vi "S4GUI.vi"(7 "Tab ObsEng":enum32{"Obs", "CCD modes", "Guider", "Eng"}(tab)) -> ()   [LabVIEW 2018] (continued)
            n1225 = call "Read Instrument.lvclass.vi"("error in (no error)"=w304, "S4ACS_GUI in"=w306) -> ("error out"=w308:errorcluster, "Instrument.lvclass"=w307:refnum<class "Instrument.lvclass">, "S4ACS_GUI out"=w296:refnum<class "S4GUI.lvclass">)  [unwired: 7 in]
            n1226 = call-dynamic "Read mode.vi"("error in (no error)"=w308, "Instrument in"=w307) -> ("error out"=w297:errorcluster, "mode"=w309:bool)  [unwired: 7 in, 1 out]
            n1227 = while {
              tunnel: w309 -> [w351]
              shift-right: [w347] -> _
              shift-left: _ -> [w350]
              shift-right: [w348] -> _
              shift-left: _ -> [w349]
              stop <- TRUE stop-if-true
              n1228 = case shown="False" w351 {
                tunnel: w350 -> [w353 w372]
                tunnel: [w354 w371] -> w347
                tunnel: w349 -> [w356 w370]
                tunnel: [w355 w369] -> w348
                frame True {
                  # "polarimetria"
                  n1229 = case shown="False" w356 {
                    selector: w356 -> [w366 w368]
                    tunnel: [w365 w368] -> w355
                    tunnel: [FALSE FALSE] -> w354
                    tunnel: w353 -> [_ _]
                    frame False {
                      w363 = 11
                      w360 = 80
                      w359 = 12900
                      # "Valor médio\ndo curso do foco."
                      n1230 = local write "Start focus"(w359) -> ()
                      n1231 = local write "Step focus"(w360) -> ()
                      n1232 = local write "#steps"(w363) -> ()
                      n1233 = Quotient & Remainder(x=w363, y=2) -> (floor(x/y)=w361:i32)  [unwired: 1 out]
                      n1234 = Multiply(x=w360, y=w361) -> (x*y=w358:i32)
                      n1235 = Add(x=w359, y=w358) -> (x+y=w357:i32)
                      n1236 = local write "Target focus 2"(w357) -> ()
                      n1237 = local write "Target focus"(w357) -> ()
                      n1238 = Not(x=w366) -> (.not. x?=w365:bool)
                    }
                    frame True {
                    }
                  }
                }
                frame False {
                  # "fotometria"
                  n1239 = case shown="False" w372 {
                    selector: w372 -> [w381 w384]
                    tunnel: [w380 w384] -> w371
                    tunnel: w370 -> [_ _]
                    tunnel: [FALSE FALSE] -> w369
                    frame False {
                      w376 = 11
                      w375 = 100
                      w374 = 13400
                      # "Valor médio\ndo curso do foco."
                      n1240 = local write "Start focus"(w374) -> ()
                      n1241 = local write "Step focus"(w375) -> ()
                      n1242 = local write "#steps"(w376) -> ()
                      n1243 = Quotient & Remainder(x=w376, y=2) -> (floor(x/y)=w378:i32)  [unwired: 1 out]
                      n1244 = Multiply(x=w375, y=w378) -> (x*y=w377:i32)
                      n1245 = Add(x=w374, y=w377) -> (x+y=w373:i32)
                      n1246 = local write "Target focus"(w373) -> ()
                      n1247 = local write "Target focus 2"(w373) -> ()
                      n1248 = Not(x=w381) -> (.not. x?=w380:bool)
                    }
                    frame True {
                    }
                  }
                }
              }
            }
            n1249 = call-dynamic "Read exit.vi"("error in (no error)"=w297, "S4GUI in"=w296) -> ("error out"=w295:errorcluster, "exit"=w294:bool, "S4GUI out"=w293:refnum<class "S4GUI.lvclass">)  [unwired: 7 in]
          }
        }
      }
      event "Lambda Selector": Mouse Down? {
        n1250 = event-data() -> ()  [unwired: 1 in, 7 out]
        n1251 = First Call?() -> (First Call?: T/F=w2000:bool)
        n1252 = case shown="True" w2000 {
          tunnel: w2002 -> [w2004 w2006]
          tunnel: [w2004 w2005] -> w2001
          frame False {
          }
          frame True {
            w2008 = u16 0 items=["OFF", "Lambda/2", "Lambda/4"] ("Lambda Selector")
            n1253 = property on="Lambda Selector" class="Ring (strict)"(error in=w2006, "Value"=w2008) -> (error out=w2009:errorcluster)  [unwired: 1 in, 1 out]
            n1254 = property on="Lambda Selector" class="Ring (strict)"(error in=w2009, "RingText.Text"="OFF" ("Boolean Text.Text")) -> (error out=w2005:errorcluster)  [unwired: 1 in, 1 out]
          }
        }
        n1255 = event-data() -> ()  [unwired: 2 in, 1 out]
      }
      event "object suffix": Key Down; "object suffix": Key Repeat {
        n1256 = event-data() -> ("Char"=w2010:i16)  [unwired: 1 in]
        "charKeyboardInteger" <- w2010
        n1257 = call-dynamic "Write charSuffix.vi"("error in (no error)"=w2013, "charSuffix"=w2010, "S4GUI in"=w2014) -> ("error out"=w2011:errorcluster, "S4GUI out"=w2012:refnum<class "S4GUI.lvclass">)  [unwired: 7 in]
      }
      event "dflat suffix": Key Down; "dflat suffix": Key Repeat {
        n1258 = event-data() -> ("Char"=w2017:i16)  [unwired: 1 in]
        n1259 = call-dynamic "Write charSuffix.vi"("error in (no error)"=w2018, "charSuffix"=w2017, "S4GUI in"=w2019) -> ("error out"=w2015:errorcluster, "S4GUI out"=w2016:refnum<class "S4GUI.lvclass">)  [unwired: 7 in]
      }
      event "sflat suffix": Key Down; "sflat suffix": Key Repeat {
        n1260 = event-data() -> ("Char"=w2022:i16)  [unwired: 1 in]
        n1261 = call-dynamic "Write charSuffix.vi"("error in (no error)"=w2023, "charSuffix"=w2022, "S4GUI in"=w2024) -> ("error out"=w2020:errorcluster, "S4GUI out"=w2021:refnum<class "S4GUI.lvclass">)  [unwired: 7 in]
      }
      event "dark suffix": Key Down; "dark suffix": Key Repeat {
        n1262 = event-data() -> ("Char"=w2027:i16)  [unwired: 1 in]
        n1263 = call-dynamic "Write charSuffix.vi"("error in (no error)"=w2028, "charSuffix"=w2027, "S4GUI in"=w2029) -> ("error out"=w2025:errorcluster, "S4GUI out"=w2026:refnum<class "S4GUI.lvclass">)  [unwired: 7 in]
      }
      event "zero suffix": Key Down; "zero suffix": Key Repeat {
        n1264 = event-data() -> ("Char"=w2032:i16)  [unwired: 1 in]
        n1265 = call-dynamic "Write charSuffix.vi"("error in (no error)"=w2033, "charSuffix"=w2032, "S4GUI in"=w2034) -> ("error out"=w2030:errorcluster, "S4GUI out"=w2031:refnum<class "S4GUI.lvclass">)  [unwired: 7 in]
      }
      event "focus suffix": Key Down; "focus suffix": Key Repeat {
        n1266 = event-data() -> ("Char"=w2037:i16)  [unwired: 1 in]
        n1267 = call-dynamic "Write charSuffix.vi"("error in (no error)"=w2038, "charSuffix"=w2037, "S4GUI in"=w2039) -> ("error out"=w2035:errorcluster, "S4GUI out"=w2036:refnum<class "S4GUI.lvclass">)  [unwired: 7 in]
      }
      event "Set CCD mode": Value Change {
        w2152 = i16 1 items=["Cooler OFF", "Cooler ON"] ("Cooler ON/OFF")
        w2166 = i16 1 items=["Cooler OFF", "Cooler ON"] ("Cooler ON/OFF")
        w2182 = i16 1 items=["Cooler OFF", "Cooler ON"] ("Cooler ON/OFF")
        w2202 = i16 1 items=["Cooler OFF", "Cooler ON"] ("Cooler ON/OFF")
        # "Sinaliza que houve requisição de SET CCD mode"
        n1268 = event-data() -> ()  [unwired: 1 in, 6 out]
        n1269 = call-dynamic "Write User Event.vi"("error in (no error)"=w2358, "User Event"="SET CCD mode ", "S4GUI in"=w2357) -> ("error out"=w2147:errorcluster, "S4GUI out"=w2146:refnum<class "S4GUI.lvclass">)  [unwired: 7 in]
        n1270 = call-dynamic "Write SET request.vi"("error in (no error)"=w2147, "SET request"=TRUE, "S4GUI in"=w2146) -> ("error out"=w2144:errorcluster, "S4GUI out"=w2145:refnum<class "S4GUI.lvclass">)  [unwired: 7 in]
        n1271 = call-dynamic "Read CCD mode.vi"("error in (no error)"=w2144, "S4GUI in"=w2145) -> ("error out"=w2355:errorcluster, "CCD mode"=w2356:T30, "S4GUI out"=w2354:refnum<class "S4GUI.lvclass">)  [unwired: 7 in]
        n1272 = Bundle By Name(cluster=w2356, "FTM"="Frame Transfer", "AQM"="AQM", "SZM"="SZM", "EM gain"="EM Gain") -> (w2353:T30)
        n1273 = call-dynamic "Write CCD mode.vi"("error in (no error)"=w2355, "CCD mode"=w2353, "S4GUI in"=w2354) -> ("error out"=w2213:errorcluster, "S4GUI out"=w2214:refnum<class "S4GUI.lvclass">)  [unwired: 7 in]
        n1274 = call-dynamic "LoadCCDmode.vi"("error in (no error)"=w2213, "S4GUI in"=w2214) -> ("error out"=w2212:errorcluster, "S4GUI out"=w2211:refnum<class "S4GUI.lvclass">)  [unwired: 8 in]
        n1275 = call-dynamic "Read Parameters CCD modes.vi"("error in (no error)"=w2212, "S4GUI in"=w2211) -> ("error out"=w2210:errorcluster, "Parameters CCD modes"=w2215:T5, "S4GUI out"=w2209:refnum<class "S4GUI.lvclass">)  [unwired: 7 in]
        n1276 = Unbundle By Name(w2215) -> ("CCD \nEM Mode"=w2345:u8, "Readout\nRate"=w2207:u8)
        n1277 = case shown="0, Default" w2345 {
          tunnel: [string[] ["30 MHz", "20 MHz", "10 MHz", "1 MHz"] ("Strings []") string[] ["1 MHz", "0.1 MHz"] ("Strings []")] -> w2346
          frame 0, Default {
          }
          frame 1 {
          }
        }
        n1278 = flat-sequence {
          tunnel: w2346 -> [w2492]
          tunnel: w2345 -> [w2493]
          tunnel: [w2493] -> w2347
          tunnel: w2215 -> [w2499]
          tunnel: [w2498] -> w2208
          tunnel: w2347 -> [w2496]
          tunnel: w2216 -> [w2497]
          tunnel: w2207 -> [w2494]
          frame #0 {
            n1279 = property on="Readout\nRate" class="Ring (strict)"("Strings []"=w2492) -> ()  [unwired: 2 in, 2 out]
            n1280 = property on="Readout\nRate" class="Ring (strict)"("Strings []"=w2492) -> ()  [unwired: 2 in, 2 out]
            n1281 = property on="Readout Rate 2" class="Ring (strict)"("Strings []"=w2492) -> ()  [unwired: 2 in, 2 out]
            n1282 = property on="Readout Rate" class="Ring (strict)"("Strings []"=w2492) -> ()  [unwired: 2 in, 2 out]
            n1283 = property on="Readout Rate 3" class="Ring (strict)"("Strings []"=w2492) -> ()  [unwired: 2 in, 2 out]
            n1284 = property on="Readout Rate 4" class="Ring (strict)"("Strings []"=w2492) -> ()  [unwired: 2 in, 2 out]
          }
          frame #1 {
            n1285 = Bundle By Name(cluster=w2499, "Readout\nRate"=w2494, "CCD \nEM Mode"=w2496) -> (w2498:T5)
            n1286 = disable-structure shown="Enabled" {
              disable-tunnel: w2497 -> [w2503 w2504]
              disable-tunnel: w2496 -> [w2502 _]
              disable-tunnel: [w2501 w2504] -> w2495
              disable-tunnel: w2494 -> [w2500 _]
              frame Disabled {
                n1287 = Bundle By Name(cluster=w2503, "Parameters.Readout\nRate"=w2500, "Parameters.CCD \nEM Mode"=w2502) -> (w2501:T8)
              }
              frame Enabled {
              }
            }
            n1288 = local write "Input Cluster"(w2495) -> ()
          }
        }
        n1289 = call-dynamic "Read InfoCCDmode.vi"("error in (no error)"=w2210, "S4GUI in"=w2209) -> ("error out"=w2348:errorcluster, "InfoCCDmode"=w2077:T2, "S4GUI out"=w2349:refnum<class "S4GUI.lvclass">)  [unwired: 7 in]
        "InfoCCDmode" <- w2077
        n1290 = Unbundle By Name(w2077) -> ("MinExpTime"=w2099:dbl)
        n1291 = call-dynamic "Read Parameters CCD modes.vi"("error in (no error)"=w2348, "S4GUI in"=w2349) -> ("error out"=w2342:errorcluster, "Parameters CCD modes"=→"Parameters CCD modes":T5, "S4GUI out"=w2343:refnum<class "S4GUI.lvclass">)  [unwired: 7 in]
        n1292 = local read "Input Cluster"() -> (w2216:T8)
        n1293 = call-dynamic "Write Parameters CCD modes.vi"("error in (no error)"=w2342, "Parameters CCD modes"=w2208, "S4GUI in"=w2343) -> ("error out"=w2321:errorcluster, "S4GUI out"=w2295:refnum<class "S4GUI.lvclass">)  [unwired: 7 in]
        n1294 = Unbundle By Name(w2208) -> ("Frame\nTransfer"=w2250:bool, "Pre-amplification\nGain"=w2249:u8, "Readout\nRate"=w2248:u8, "CCD \nEM Mode"=w2247:u8, "CCD\nEM Gain"=w2246:u16, "Image \nInitial Line"=w2245:u16, "Image\nInitial Column"=w2244:u16, "Image\nFinal Line"=w2234:u16, "Image\nFInal Column"=w2243:u16, "Vertical\nBinning"=w2242:u16, "Horizontal\nBinning"=w2241:u16)
        n1295 = call-dynamic "Read AcquisitionA.vi"("error in (no error)"=w2321, "S4ACS_GUI in"=w2295) -> ("error out"=w2232:errorcluster, "Acquisition.lvclass"=w2233:refnum<class "Acquisition.lvclass">, "S4ACS_GUI out"=w2341:refnum<class "S4GUI.lvclass">)  [unwired: 7 in]
        n1296 = call-dynamic "Read enabled.vi"("error in (no error)"=w2232, "Server in"=w2233) -> ("error out"=w2231:errorcluster, "enabled"=w2229:bool, "Server out"=w2230:refnum<class "Acquisition.lvclass">)  [unwired: 7 in]
        n1297 = call-dynamic "Read Channel.vi"("error in (no error)"=w2231, "Acquisition in"=w2230) -> ("error out"=w2338:errorcluster, "Channel.lvclass"=w2339:refnum<class "Channel.lvclass">, "Acquisition out"=w2340:refnum<class "Acquisition.lvclass">)  [unwired: 7 in]
        n1298 = call-dynamic "Read Interface.vi"("error in (no error)"=w2338, "Channel in"=w2339) -> ("error out"=w2324:errorcluster, "Interface.lvclass"=w2325:refnum<class "Interface.lvclass">, "Channel out"=w2319:refnum<class "Channel.lvclass">)  [unwired: 7 in]
        n1299 = call-dynamic "Write PREV_FT.vi"("error in (no error)"=w2324, "PREV_FT"=w2250, "Interface in"=w2325) -> ("error out"=w2205:errorcluster, "Interface out"=w2204:refnum<class "Interface.lvclass">)  [unwired: 7 in]
        n1300 = call-dynamic "Write Cooler ON_OFF.vi"("error in (no error)"=w2205, "Cooler ON/OFF"=w2202, "Interface in"=w2204) -> ("error out"=w2203:errorcluster, "Interface out"=w2201:refnum<class "Interface.lvclass">)  [unwired: 7 in]
        n1301 = call-dynamic "Read target cluster.vi"("error in (no error)"=w2203, "Channel in"=w2319) -> ("error out"=w2317:errorcluster, "target cluster"=w2316:T31, "Channel out"=w2318:refnum<class "Channel.lvclass">)  [unwired: 7 in]
        n1302 = Bundle By Name(cluster=w2316, "FRAME_TRANSFER"=w2250, "PREAMP"=w2249, "READOUT_RATE"=w2248, "EM_MODE"=w2247, "EM_GAIN"=w2246, "INITIAL_LINE"=w2245, "INITIAL_COLUMN"=w2244, "FINAL_LINE"=w2234, "FINAL_COLUMN"=w2243, "VBIN"=w2242, "HBIN"=w2241) -> (w2198:T31)
        n1303 = call-dynamic "Write target cluster.vi"("error in (no error)"=w2317, "target cluster"=w2198, "Channel in"=w2318) -> ("error out"=w2199:errorcluster, "Channel out"=w2323:refnum<class "Channel.lvclass">)  [unwired: 7 in]
        n1304 = call-dynamic "Set CCD_Config.vi"("error in (no error)"=w2199, "input cluster"=w2198, "Interface in"=w2201) -> ("error out"=w2188:errorcluster, "Interface out"=w2200:refnum<class "Interface.lvclass">)  [unwired: 7 in]
        n1305 = Flatten To String(anything=w2198, error in (no error)=w2199) -> (data string=w2333:string)  [unwired: 2 in, 2 out]
        n1306 = call "Write flatted cluster.vi"("error in (no error)"=w2188, "flatted cluster"=w2333, "Interface in"=w2200) -> ("error out"=w2138:errorcluster, "Interface out"=w2139:refnum<class "Interface.lvclass">)  [unwired: 7 in]
        n1307 = call "Read Exposure Time.vi"("error in (no error)"=w2138, "Interface in"=w2139) -> ("error out"=w2136:errorcluster, "Exposure Time"=w2141:dbl, "Interface out"=w2137:refnum<class "Interface.lvclass">)  [unwired: 7 in]
        n1308 = Greater Or Equal?(x=w2141, y=w2099) -> (x >= y?=w2142:bool)
        n1309 = Select(t=w2141, s=w2142, f=w2099) -> (s? t:f=w2140:dbl)
        n1310 = local write "Exptime ch1"(w2140) -> ()
        n1311 = call "Write Exposure Time.vi"("error in (no error)"=w2136, "Exposure Time"=w2140, "Interface in"=w2137) -> ("error out"=w2097:errorcluster, "Interface out"=w2098:refnum<class "Interface.lvclass">)  [unwired: 7 in]
        n1312 = call-dynamic "ValidateExp.vi"("error in (no error)"=w2097, "Interface in"=w2098) -> ("error out"=w2080:errorcluster, "Interface out"=w2082:refnum<class "Interface.lvclass">)  [unwired: 8 in]
        n1313 = call-dynamic "Read MAX #FRAMES.vi"("error in (no error)"=w2080, "Interface in"=w2082) -> ("error out"=w2079:errorcluster, "MAX #FRAMES"=w2076:u32, "Interface out"=w2081:refnum<class "Interface.lvclass">)  [unwired: 7 in]
        n1314 = call-dynamic "Read # Images.vi"("error in (no error)"=w2079, "Interface in"=w2081) -> ("error out"=w2095:errorcluster, "# Images"=w2083:u32, "Interface out"=w2096:refnum<class "Interface.lvclass">)  [unwired: 7 in]
        n1315 = call-dynamic "Write #PREV Images.vi"("error in (no error)"=w2095, "#PREV FRAMES"=w2083, "Interface in"=w2096) -> ("error out"=w2093:errorcluster, "Interface out"=w2094:refnum<class "Interface.lvclass">)  [unwired: 7 in]
        n1316 = call-dynamic "Write Interface.vi"("error in (no error)"=w2093, "Interface.lvclass"=w2094, "Channel in"=w2323) -> ("error out"=w2329:errorcluster, "Channel out"=w2331:refnum<class "Channel.lvclass">)  [unwired: 7 in]
        n1317 = local write "Exp ch1"(w2083) -> ()
        n1318 = property on="Exposures Done ch1" class="Slide (strict)"("Scale.Maximum"=w2083, "Scale.Minimum"=0.0 ("Scale.Range:Minimum")) -> ()  [unwired: 2 in, 2 out]
        n1319 = call "Write section_name.vi"("error in (no error)"=w2329, "section_name"="CCD_ACS1", "Channel in"=w2331) -> ("error out"=w2328:errorcluster, "Channel out"=w2330:refnum<class "Channel.lvclass">)  [unwired: 7 in]
        n1320 = call-dynamic "save config.vi"("error in (no error)"=w2328, "file config"="lastsaved.cfg", "Channel in"=w2330) -> ("error out"=w2196:errorcluster, "Channel out"=w2197:refnum<class "Channel.lvclass">)  [unwired: 7 in]
        n1321 = call-dynamic "ValidateConfig.vi"("error in (no error)"=w2196, "Channel in"=w2197) -> ("error out"=w2194:errorcluster, "Channel out"=w2195:refnum<class "Channel.lvclass">)  [unwired: 7 in, 1 out]
        n1322 = call-dynamic "Save Temp.vi"("error in (no error)"=w2194, "temp file"="lasttemp.cfg" ("file config"), "Channel in"=w2195) -> ("error out"=w2193:errorcluster, "Channel out"=w2192:refnum<class "Channel.lvclass">)  [unwired: 7 in]
        n1323 = case shown="True" w2229 {
          tunnel: [w2460 w2485] -> w2337
          tunnel: [w2459 w2484] -> w2336
          tunnel: w2192 -> [w2460 w2483]
          tunnel: w2193 -> [w2459 w2482]
          frame False {
          }
          frame True {
            # "Esvazia\na fila."
            n1324 = call-dynamic "Read State Machine.vi"("error in (no error)"=w2482, "Device in"=w2483) -> ("error out"=w2476:errorcluster, "State Machine.lvclass"=w2479:refnum<class "State Machine.lvclass">, "Device out"=w2489:refnum<class "Channel.lvclass">)  [unwired: 7 in]
            n1325 = call-dynamic "Read ref StatesQueue.vi"("error in (no error)"=w2476, "State Machine in"=w2479) -> ("error out"=w2467:errorcluster, "ref StatesQueue"=w2469:refnum<queue>, "State Machine out"=w2478:refnum<class "State Machine.lvclass">)  [unwired: 7 in]
            n1326 = Flush Queue(queue=w2469, error in (no error)=w2467) -> (queue out=w2468:refnum<queue>, error out=w2466:errorcluster)  [unwired: 1 out]
            n1327 = Enqueue Element(queue=w2468, element=u32 60 ("State"), error in (no error)=w2466) -> (queue out=w2481:refnum<queue>, error out=w2475:errorcluster)  [unwired: 1 in, 1 out]
            n1328 = Enqueue Element(queue=w2481, element=u32 45 ("State"), error in (no error)=w2475) -> (queue out=w2480:refnum<queue>, error out=w2474:errorcluster)  [unwired: 1 in, 1 out]
            n1329 = Enqueue Element(queue=w2480, element=u32 35 ("State"), error in (no error)=w2474) -> (queue out=w2464:refnum<queue>, error out=w2463:errorcluster)  [unwired: 1 in, 1 out]
            n1330 = Enqueue Element(queue=w2464, element=u32 37 ("State"), error in (no error)=w2463) -> (queue out=w2461:refnum<queue>, error out=w2462:errorcluster)  [unwired: 1 in, 1 out]
            n1331 = call-dynamic "Write ref StatesQueue.vi"("error in (no error)"=w2462, "ref StatesQueue"=w2461, "State Machine in"=w2478) -> ("error out"=w2470:errorcluster, "State Machine out"=w2477:refnum<class "State Machine.lvclass">)  [unwired: 7 in]
            n1332 = disable-structure shown="Enabled" {
              disable-tunnel: [0 ("State") 45] -> w2486
              frame Enabled {
                # "Vai pra 0 para que\nos estados da fila \nsejam retirados."
              }
              frame Disabled {
                # "Verifica Texp\nantes de tudo."
              }
            }
            n1333 = call-dynamic "Write State.vi"("error in (no error)"=w2470, "State"=w2486, "State Machine in"=w2477) -> ("error out"=w2487:errorcluster, "State Machine out"=w2488:refnum<class "State Machine.lvclass">)  [unwired: 7 in]
            n1334 = call-dynamic "Write State Machine.vi"("error in (no error)"=w2487, "State Machine.lvclass"=w2488, "Device in"=w2489) -> ("error out"=w2484:errorcluster, "Device out"=w2485:refnum<class "Channel.lvclass">)  [unwired: 7 in]
          }
        }
        n1335 = Bundle By Name(cluster=w2077, "MaxExp"=w2076) -> (w2078:T2)
        n1336 = call-dynamic "Write Channel.vi"("error in (no error)"=w2336, "Channel.lvclass"=w2337, "Acquisition in"=w2340) -> ("error out"=w2335:errorcluster, "Acquisition out"=w2334:refnum<class "Acquisition.lvclass">)  [unwired: 7 in]
        n1337 = local write "InfoCCDmode"(w2078) -> ()
        n1338 = call-dynamic "Write AcquisitionA.vi"("error in (no error)"=w2335, "Acquisition.lvclass"=w2334, "S4ACS_GUI in"=w2341) -> ("error out"=w2090:errorcluster, "S4ACS_GUI out"=w2091:refnum<class "S4GUI.lvclass">)  [unwired: 7 in]
        n1339 = call-dynamic "Read InfoCCDmode.vi"("error in (no error)"=w2090, "S4GUI in"=w2091) -> ("error out"=w2088:errorcluster, "InfoCCDmode"=w2087:T2, "S4GUI out"=w2089:refnum<class "S4GUI.lvclass">)  [unwired: 7 in]
        n1340 = Bundle By Name(cluster=w2087, "MaxExp"=w2076) -> (w2086:T2)
        n1341 = call-dynamic "Write InfoCCDmode.vi"("error in (no error)"=w2088, "InfoCCDmode"=w2086, "S4GUI in"=w2089) -> ("error out"=w2084:errorcluster, "S4GUI out"=w2085:refnum<class "S4GUI.lvclass">)  [unwired: 7 in]
        n1342 = call "Read AcquisitionB.vi"("error in (no error)"=errorcluster {"status"=FALSE, "code"=0, "source"=""}, "S4ACS_GUI in"=w2085) -> ("error out"=w2225:errorcluster, "Acquisition.lvclass"=w2228:refnum<class "Acquisition.lvclass">, "S4ACS_GUI out"=w2315:refnum<class "S4GUI.lvclass">)  [unwired: 7 in]
        n1343 = call-dynamic "Read enabled.vi"("error in (no error)"=w2225, "Server in"=w2228) -> ("error out"=w2226:errorcluster, "enabled"=w2121:bool, "Server out"=w2227:refnum<class "Acquisition.lvclass">)  [unwired: 7 in]
        n1344 = call-dynamic "Read Channel.vi"("error in (no error)"=w2226, "Acquisition in"=w2227) -> ("error out"=w2312:errorcluster, "Channel.lvclass"=w2313:refnum<class "Channel.lvclass">, "Acquisition out"=w2314:refnum<class "Acquisition.lvclass">)  [unwired: 7 in]
        n1345 = call-dynamic "Read Interface.vi"("error in (no error)"=w2312, "Channel in"=w2313) -> ("error out"=w2301:errorcluster, "Interface.lvclass"=w2302:refnum<class "Interface.lvclass">, "Channel out"=w2299:refnum<class "Channel.lvclass">)  [unwired: 7 in]
        n1346 = call-dynamic "Write PREV_FT.vi"("error in (no error)"=w2301, "PREV_FT"=w2250, "Interface in"=w2302) -> ("error out"=w2183:errorcluster, "Interface out"=w2185:refnum<class "Interface.lvclass">)  [unwired: 7 in]
        n1347 = call-dynamic "Write Cooler ON_OFF.vi"("error in (no error)"=w2183, "Cooler ON/OFF"=w2182, "Interface in"=w2185) -> ("error out"=w2181:errorcluster, "Interface out"=w2184:refnum<class "Interface.lvclass">)  [unwired: 7 in]
        n1348 = call-dynamic "Read target cluster.vi"("error in (no error)"=w2181, "Channel in"=w2299) -> ("error out"=w2297:errorcluster, "target cluster"=w2296:T31, "Channel out"=w2298:refnum<class "Channel.lvclass">)  [unwired: 7 in]
        n1349 = Bundle By Name(cluster=w2296, "FRAME_TRANSFER"=w2250, "PREAMP"=w2249, "READOUT_RATE"=w2248, "EM_MODE"=w2247, "EM_GAIN"=w2246, "INITIAL_LINE"=w2245, "INITIAL_COLUMN"=w2244, "FINAL_LINE"=w2234, "FINAL_COLUMN"=w2243, "VBIN"=w2242, "HBIN"=w2241) -> (w2186:T31)
        n1350 = call-dynamic "Write target cluster.vi"("error in (no error)"=w2297, "target cluster"=w2186, "Channel in"=w2298) -> ("error out"=w2189:errorcluster, "Channel out"=w2300:refnum<class "Channel.lvclass">)  [unwired: 7 in]
        n1351 = call-dynamic "Set CCD_Config.vi"("error in (no error)"=w2189, "input cluster"=w2186, "Interface in"=w2184) -> ("error out"=w2187:errorcluster, "Interface out"=w2190:refnum<class "Interface.lvclass">)  [unwired: 7 in]
        n1352 = Flatten To String(anything=w2186, error in (no error)=w2189) -> (data string=w2309:string)  [unwired: 2 in, 2 out]
        n1353 = call "Write flatted cluster.vi"("error in (no error)"=w2187, "flatted cluster"=w2309, "Interface in"=w2190) -> ("error out"=w2114:errorcluster, "Interface out"=w2115:refnum<class "Interface.lvclass">)  [unwired: 7 in]
        n1354 = call "Read Exposure Time.vi"("error in (no error)"=w2114, "Interface in"=w2115) -> ("error out"=w2135:errorcluster, "Exposure Time"=w2116:dbl, "Interface out"=w2134:refnum<class "Interface.lvclass">)  [unwired: 7 in]
        n1355 = Greater Or Equal?(x=w2116, y=w2099) -> (x >= y?=w2132:bool)
        n1356 = Select(t=w2116, s=w2132, f=w2099) -> (s? t:f=w2133:dbl)
        n1357 = local write "Exptime ch2"(w2133) -> ()
        n1358 = call "Write Exposure Time.vi"("error in (no error)"=w2135, "Exposure Time"=w2133, "Interface in"=w2134) -> ("error out"=w2061:errorcluster, "Interface out"=w2066:refnum<class "Interface.lvclass">)  [unwired: 7 in]
        n1359 = call-dynamic "ValidateExp.vi"("error in (no error)"=w2061, "Interface in"=w2066) -> ("error out"=w2074:errorcluster, "Interface out"=w2065:refnum<class "Interface.lvclass">)  [unwired: 8 in]
        n1360 = call-dynamic "Read MAX #FRAMES.vi"("error in (no error)"=w2074, "Interface in"=w2065) -> ("error out"=w2075:errorcluster, "Interface out"=w2064:refnum<class "Interface.lvclass">)  [unwired: 7 in, 1 out]
        n1361 = call-dynamic "Read # Images.vi"("error in (no error)"=w2075, "Interface in"=w2064) -> ("error out"=w2073:errorcluster, "# Images"=w2058:u32, "Interface out"=w2063:refnum<class "Interface.lvclass">)  [unwired: 7 in]
        n1362 = call-dynamic "Write #PREV Images.vi"("error in (no error)"=w2073, "#PREV FRAMES"=w2058, "Interface in"=w2063) -> ("error out"=w2060:errorcluster, "Interface out"=w2062:refnum<class "Interface.lvclass">)  [unwired: 7 in]
        n1363 = local write "Exp ch2"(w2058) -> ()
        n1364 = property on="Exposures Done ch2" class="Slide (strict)"("Scale.Maximum"=w2058, "Scale.Minimum"=0.0 ("Scale.Range:Minimum")) -> ()  [unwired: 2 in, 2 out]
        n1365 = call-dynamic "Write Interface.vi"("error in (no error)"=w2060, "Interface.lvclass"=w2062, "Channel in"=w2300) -> ("error out"=w2305:errorcluster, "Channel out"=w2307:refnum<class "Channel.lvclass">)  [unwired: 7 in]
        n1366 = call "Write section_name.vi"("error in (no error)"=w2305, "section_name"="CCD_ACS2", "Channel in"=w2307) -> ("error out"=w2304:errorcluster, "Channel out"=w2306:refnum<class "Channel.lvclass">)  [unwired: 7 in]
        n1367 = call-dynamic "save config.vi"("error in (no error)"=w2304, "file config"="lastsaved.cfg", "Channel in"=w2306) -> ("error out"=w2176:errorcluster, "Channel out"=w2177:refnum<class "Channel.lvclass">)  [unwired: 7 in]
        n1368 = call-dynamic "ValidateConfig.vi"("error in (no error)"=w2176, "Channel in"=w2177) -> ("error out"=w2179:errorcluster, "Channel out"=w2180:refnum<class "Channel.lvclass">)  [unwired: 7 in, 1 out]
        n1369 = call-dynamic "Save Temp.vi"("error in (no error)"=w2179, "temp file"="lasttemp.cfg" ("file config"), "Channel in"=w2180) -> ("error out"=w2119:errorcluster, "Channel out"=w2120:refnum<class "Channel.lvclass">)  [unwired: 7 in]
        n1370 = case shown="True" w2121 {
          tunnel: [w2394 w2419] -> w2118
          tunnel: [w2393 w2418] -> w2117
          tunnel: w2120 -> [w2394 w2417]
          tunnel: w2119 -> [w2393 w2416]
          frame False {
          }
          frame True {
            # "Esvazia\na fila."
            n1371 = call-dynamic "Read State Machine.vi"("error in (no error)"=w2416, "Device in"=w2417) -> ("error out"=w2410:errorcluster, "State Machine.lvclass"=w2413:refnum<class "State Machine.lvclass">, "Device out"=w2423:refnum<class "Channel.lvclass">)  [unwired: 7 in]
            n1372 = call-dynamic "Read ref StatesQueue.vi"("error in (no error)"=w2410, "State Machine in"=w2413) -> ("error out"=w2400:errorcluster, "ref StatesQueue"=w2402:refnum<queue>, "State Machine out"=w2412:refnum<class "State Machine.lvclass">)  [unwired: 7 in]
            n1373 = Flush Queue(queue=w2402, error in (no error)=w2400) -> (queue out=w2401:refnum<queue>, error out=w2399:errorcluster)  [unwired: 1 out]
            n1374 = Enqueue Element(queue=w2401, element=u32 60 ("State"), error in (no error)=w2399) -> (queue out=w2415:refnum<queue>, error out=w2409:errorcluster)  [unwired: 1 in, 1 out]
            n1375 = Enqueue Element(queue=w2415, element=u32 45 ("State"), error in (no error)=w2409) -> (queue out=w2414:refnum<queue>, error out=w2408:errorcluster)  [unwired: 1 in, 1 out]
            n1376 = Enqueue Element(queue=w2414, element=u32 35 ("State"), error in (no error)=w2408) -> (queue out=w2407:refnum<queue>, error out=w2397:errorcluster)  [unwired: 1 in, 1 out]
            n1377 = Enqueue Element(queue=w2407, element=u32 37, error in (no error)=w2397) -> (queue out=w2398:refnum<queue>, error out=w2396:errorcluster)  [unwired: 1 in, 1 out]
            n1378 = call-dynamic "Write ref StatesQueue.vi"("error in (no error)"=w2396, "ref StatesQueue"=w2398, "State Machine in"=w2412) -> ("error out"=w2403:errorcluster, "State Machine out"=w2411:refnum<class "State Machine.lvclass">)  [unwired: 7 in]
            n1379 = disable-structure shown="Enabled" {
              disable-tunnel: [0 ("State") 45] -> w2420
              frame Enabled {
                # "Vai pra 0 para que\nos estados da fila \nsejam retirados."
              }
              frame Disabled {
                # "Verifica Texp\nantes de tudo."
              }
            }
            n1380 = call-dynamic "Write State.vi"("error in (no error)"=w2403, "State"=w2420, "State Machine in"=w2411) -> ("error out"=w2421:errorcluster, "State Machine out"=w2422:refnum<class "State Machine.lvclass">)  [unwired: 7 in]
            n1381 = call-dynamic "Write State Machine.vi"("error in (no error)"=w2421, "State Machine.lvclass"=w2422, "Device in"=w2423) -> ("error out"=w2418:errorcluster, "Device out"=w2419:refnum<class "Channel.lvclass">)  [unwired: 7 in]
          }
        }
        n1382 = call-dynamic "Write Channel.vi"("error in (no error)"=w2117, "Channel.lvclass"=w2118, "Acquisition in"=w2314) -> ("error out"=w2311:errorcluster, "Acquisition out"=w2310:refnum<class "Acquisition.lvclass">)  [unwired: 7 in]
        n1383 = call "Write AcquisitionB.vi"("error in (no error)"=w2311, "Acquisition.lvclass"=w2310, "S4ACS_GUI in"=w2315) -> ("error out"=w2238:errorcluster, "S4ACS_GUI out"=w2272:refnum<class "S4GUI.lvclass">)  [unwired: 7 in]
        n1384 = call-dynamic "Read AcquisitionC.vi"("error in (no error)"=errorcluster {"status"=FALSE, "code"=0, "source"=""}, "S4ACS_GUI in"=w2272) -> ("error out"=w2222:errorcluster, "Acquisition.lvclass"=w2224:refnum<class "Acquisition.lvclass">, "S4ACS_GUI out"=w2293:refnum<class "S4GUI.lvclass">)  [unwired: 7 in]
        n1385 = call-dynamic "Read enabled.vi"("error in (no error)"=w2222, "Server in"=w2224) -> ("error out"=w2221:errorcluster, "enabled"=w2113:bool, "Server out"=w2223:refnum<class "Acquisition.lvclass">)  [unwired: 7 in]
        n1386 = call-dynamic "Read Channel.vi"("error in (no error)"=w2221, "Acquisition in"=w2223) -> ("error out"=w2290:errorcluster, "Channel.lvclass"=w2291:refnum<class "Channel.lvclass">, "Acquisition out"=w2292:refnum<class "Acquisition.lvclass">)  [unwired: 7 in]
        n1387 = call-dynamic "Read Interface.vi"("error in (no error)"=w2290, "Channel in"=w2291) -> ("error out"=w2279:errorcluster, "Interface.lvclass"=w2280:refnum<class "Interface.lvclass">, "Channel out"=w2277:refnum<class "Channel.lvclass">)  [unwired: 7 in]
        n1388 = call-dynamic "Write PREV_FT.vi"("error in (no error)"=w2279, "PREV_FT"=w2250, "Interface in"=w2280) -> ("error out"=w2163:errorcluster, "Interface out"=w2165:refnum<class "Interface.lvclass">)  [unwired: 7 in]
        n1389 = call-dynamic "Write Cooler ON_OFF.vi"("error in (no error)"=w2163, "Cooler ON/OFF"=w2166, "Interface in"=w2165) -> ("error out"=w2162:errorcluster, "Interface out"=w2164:refnum<class "Interface.lvclass">)  [unwired: 7 in]
        n1390 = call-dynamic "Read target cluster.vi"("error in (no error)"=w2162, "Channel in"=w2277) -> ("error out"=w2275:errorcluster, "target cluster"=w2274:T31, "Channel out"=w2276:refnum<class "Channel.lvclass">)  [unwired: 7 in]
        n1391 = Bundle By Name(cluster=w2274, "FRAME_TRANSFER"=w2250, "PREAMP"=w2249, "READOUT_RATE"=w2248, "EM_MODE"=w2247, "EM_GAIN"=w2246, "INITIAL_LINE"=w2245, "INITIAL_COLUMN"=w2244, "FINAL_LINE"=w2234, "FINAL_COLUMN"=w2243, "VBIN"=w2242, "HBIN"=w2241) -> (w2170:T31)
        n1392 = call-dynamic "Write target cluster.vi"("error in (no error)"=w2275, "target cluster"=w2170, "Channel in"=w2276) -> ("error out"=w2169:errorcluster, "Channel out"=w2278:refnum<class "Channel.lvclass">)  [unwired: 7 in]
        n1393 = call-dynamic "Set CCD_Config.vi"("error in (no error)"=w2169, "input cluster"=w2170, "Interface in"=w2164) -> ("error out"=w2168:errorcluster, "Interface out"=w2167:refnum<class "Interface.lvclass">)  [unwired: 7 in]
        n1394 = Flatten To String(anything=w2170, error in (no error)=w2169) -> (data string=w2287:string)  [unwired: 2 in, 2 out]
        n1395 = call "Write flatted cluster.vi"("error in (no error)"=w2168, "flatted cluster"=w2287, "Interface in"=w2167) -> ("error out"=w2107:errorcluster, "Interface out"=w2108:refnum<class "Interface.lvclass">)  [unwired: 7 in]
        n1396 = call "Read Exposure Time.vi"("error in (no error)"=w2107, "Interface in"=w2108) -> ("error out"=w2127:errorcluster, "Exposure Time"=w2130:dbl, "Interface out"=w2128:refnum<class "Interface.lvclass">)  [unwired: 7 in]
        n1397 = Greater Or Equal?(x=w2130, y=w2099) -> (x >= y?=w2131:bool)
        n1398 = Select(t=w2130, s=w2131, f=w2099) -> (s? t:f=w2129:dbl)
        n1399 = local write "Exptime ch3"(w2129) -> ()
        n1400 = call "Write Exposure Time.vi"("error in (no error)"=w2127, "Exposure Time"=w2129, "Interface in"=w2128) -> ("error out"=w2052:errorcluster, "Interface out"=w2057:refnum<class "Interface.lvclass">)  [unwired: 7 in]
        n1401 = call-dynamic "ValidateExp.vi"("error in (no error)"=w2052, "Interface in"=w2057) -> ("error out"=w2071:errorcluster, "Interface out"=w2056:refnum<class "Interface.lvclass">)  [unwired: 8 in]
        n1402 = call-dynamic "Read MAX #FRAMES.vi"("error in (no error)"=w2071, "Interface in"=w2056) -> ("error out"=w2070:errorcluster, "Interface out"=w2055:refnum<class "Interface.lvclass">)  [unwired: 7 in, 1 out]
        n1403 = call-dynamic "Read # Images.vi"("error in (no error)"=w2070, "Interface in"=w2055) -> ("error out"=w2072:errorcluster, "# Images"=w2049:u32, "Interface out"=w2054:refnum<class "Interface.lvclass">)  [unwired: 7 in]
        n1404 = call-dynamic "Write #PREV Images.vi"("error in (no error)"=w2072, "#PREV FRAMES"=w2049, "Interface in"=w2054) -> ("error out"=w2051:errorcluster, "Interface out"=w2053:refnum<class "Interface.lvclass">)  [unwired: 7 in]
        n1405 = local write "Exp ch3"(w2049) -> ()
        n1406 = property on="Exposures Done ch3" class="Slide (strict)"("Scale.Maximum"=w2049, "Scale.Minimum"=0.0 ("Scale.Range:Minimum")) -> ()  [unwired: 2 in, 2 out]
        n1407 = call-dynamic "Write Interface.vi"("error in (no error)"=w2051, "Interface.lvclass"=w2053, "Channel in"=w2278) -> ("error out"=w2283:errorcluster, "Channel out"=w2285:refnum<class "Channel.lvclass">)  [unwired: 7 in]
        n1408 = call "Write section_name.vi"("error in (no error)"=w2283, "section_name"="CCD_ACS3", "Channel in"=w2285) -> ("error out"=w2282:errorcluster, "Channel out"=w2284:refnum<class "Channel.lvclass">)  [unwired: 7 in]
        n1409 = call-dynamic "save config.vi"("error in (no error)"=w2282, "file config"="lastsaved.cfg", "Channel in"=w2284) -> ("error out"=w2171:errorcluster, "Channel out"=w2172:refnum<class "Channel.lvclass">)  [unwired: 7 in]
        n1410 = call-dynamic "ValidateConfig.vi"("error in (no error)"=w2171, "Channel in"=w2172) -> ("error out"=w2174:errorcluster, "Channel out"=w2175:refnum<class "Channel.lvclass">)  [unwired: 7 in, 1 out]
        n1411 = call-dynamic "Save Temp.vi"("error in (no error)"=w2174, "temp file"="lasttemp.cfg" ("file config"), "Channel in"=w2175) -> ("error out"=w2111:errorcluster, "Channel out"=w2112:refnum<class "Channel.lvclass">)  [unwired: 7 in]
        n1412 = case shown="True" w2113 {
          tunnel: [w2361 w2386] -> w2110
          tunnel: [w2360 w2385] -> w2109
          tunnel: w2112 -> [w2361 w2384]
          tunnel: w2111 -> [w2360 w2383]
          frame False {
          }
          frame True {
            # "Esvazia\na fila."
            n1413 = call-dynamic "Read State Machine.vi"("error in (no error)"=w2383, "Device in"=w2384) -> ("error out"=w2377:errorcluster, "State Machine.lvclass"=w2380:refnum<class "State Machine.lvclass">, "Device out"=w2390:refnum<class "Channel.lvclass">)  [unwired: 7 in]
            n1414 = call-dynamic "Read ref StatesQueue.vi"("error in (no error)"=w2377, "State Machine in"=w2380) -> ("error out"=w2367:errorcluster, "ref StatesQueue"=w2369:refnum<queue>, "State Machine out"=w2379:refnum<class "State Machine.lvclass">)  [unwired: 7 in]
            n1415 = Flush Queue(queue=w2369, error in (no error)=w2367) -> (queue out=w2368:refnum<queue>, error out=w2366:errorcluster)  [unwired: 1 out]
            n1416 = Enqueue Element(queue=w2368, element=u32 60 ("State"), error in (no error)=w2366) -> (queue out=w2382:refnum<queue>, error out=w2376:errorcluster)  [unwired: 1 in, 1 out]
            n1417 = Enqueue Element(queue=w2382, element=u32 45 ("State"), error in (no error)=w2376) -> (queue out=w2381:refnum<queue>, error out=w2375:errorcluster)  [unwired: 1 in, 1 out]
            n1418 = Enqueue Element(queue=w2381, element=u32 35 ("State"), error in (no error)=w2375) -> (queue out=w2374:refnum<queue>, error out=w2364:errorcluster)  [unwired: 1 in, 1 out]
            n1419 = Enqueue Element(queue=w2374, element=u32 37, error in (no error)=w2364) -> (queue out=w2365:refnum<queue>, error out=w2363:errorcluster)  [unwired: 1 in, 1 out]
            n1420 = call-dynamic "Write ref StatesQueue.vi"("error in (no error)"=w2363, "ref StatesQueue"=w2365, "State Machine in"=w2379) -> ("error out"=w2370:errorcluster, "State Machine out"=w2378:refnum<class "State Machine.lvclass">)  [unwired: 7 in]
            n1421 = disable-structure shown="Enabled" {
              disable-tunnel: [0 ("State") 45] -> w2387
              frame Enabled {
                # "Vai pra 0 para que\nos estados da fila \nsejam retirados."
              }
              frame Disabled {
                # "Verifica Texp\nantes de tudo."
              }
            }
            n1422 = call-dynamic "Write State.vi"("error in (no error)"=w2370, "State"=w2387, "State Machine in"=w2378) -> ("error out"=w2388:errorcluster, "State Machine out"=w2389:refnum<class "State Machine.lvclass">)  [unwired: 7 in]
            n1423 = call-dynamic "Write State Machine.vi"("error in (no error)"=w2388, "State Machine.lvclass"=w2389, "Device in"=w2390) -> ("error out"=w2385:errorcluster, "Device out"=w2386:refnum<class "Channel.lvclass">)  [unwired: 7 in]
          }
        }
        n1424 = call-dynamic "Write Channel.vi"("error in (no error)"=w2109, "Channel.lvclass"=w2110, "Acquisition in"=w2292) -> ("error out"=w2289:errorcluster, "Acquisition out"=w2288:refnum<class "Acquisition.lvclass">)  [unwired: 7 in]
        n1425 = call-dynamic "Write AcquisitionC.vi"("error in (no error)"=w2289, "Acquisition.lvclass"=w2288, "S4ACS_GUI in"=w2293) -> ("error out"=w2237:errorcluster, "S4ACS_GUI out"=w2240:refnum<class "S4GUI.lvclass">)  [unwired: 7 in]
        n1426 = call-dynamic "Read AcquisitionD.vi"("error in (no error)"=errorcluster {"status"=FALSE, "code"=0, "source"=""}, "S4ACS_GUI in"=w2240) -> ("error out"=w2218:errorcluster, "Acquisition.lvclass"=w2220:refnum<class "Acquisition.lvclass">, "S4ACS_GUI out"=w2271:refnum<class "S4GUI.lvclass">)  [unwired: 7 in]
        n1427 = call-dynamic "Read enabled.vi"("error in (no error)"=w2218, "Server in"=w2220) -> ("error out"=w2217:errorcluster, "enabled"=w2106:bool, "Server out"=w2219:refnum<class "Acquisition.lvclass">)  [unwired: 7 in]
        n1428 = call-dynamic "Read Channel.vi"("error in (no error)"=w2217, "Acquisition in"=w2219) -> ("error out"=w2268:errorcluster, "Channel.lvclass"=w2269:refnum<class "Channel.lvclass">, "Acquisition out"=w2270:refnum<class "Acquisition.lvclass">)  [unwired: 7 in]
        n1429 = call-dynamic "Read Interface.vi"("error in (no error)"=w2268, "Channel in"=w2269) -> ("error out"=w2257:errorcluster, "Interface.lvclass"=w2258:refnum<class "Interface.lvclass">, "Channel out"=w2255:refnum<class "Channel.lvclass">)  [unwired: 7 in]
        n1430 = call-dynamic "Write PREV_FT.vi"("error in (no error)"=w2257, "PREV_FT"=w2250, "Interface in"=w2258) -> ("error out"=w2151:errorcluster, "Interface out"=w2150:refnum<class "Interface.lvclass">)  [unwired: 7 in]
        n1431 = call-dynamic "Write Cooler ON_OFF.vi"("error in (no error)"=w2151, "Cooler ON/OFF"=w2152, "Interface in"=w2150) -> ("error out"=w2148:errorcluster, "Interface out"=w2149:refnum<class "Interface.lvclass">)  [unwired: 7 in]
        n1432 = call-dynamic "Read target cluster.vi"("error in (no error)"=w2148, "Channel in"=w2255) -> ("error out"=w2253:errorcluster, "target cluster"=w2252:T31, "Channel out"=w2254:refnum<class "Channel.lvclass">)  [unwired: 7 in]
        n1433 = Bundle By Name(cluster=w2252, "FRAME_TRANSFER"=w2250, "PREAMP"=w2249, "READOUT_RATE"=w2248, "EM_MODE"=w2247, "EM_GAIN"=w2246, "INITIAL_LINE"=w2245, "INITIAL_COLUMN"=w2244, "FINAL_LINE"=w2234, "FINAL_COLUMN"=w2243, "VBIN"=w2242, "HBIN"=w2241) -> (w2153:T31)
        n1434 = call-dynamic "Write target cluster.vi"("error in (no error)"=w2253, "target cluster"=w2153, "Channel in"=w2254) -> ("error out"=w2154:errorcluster, "Channel out"=w2256:refnum<class "Channel.lvclass">)  [unwired: 7 in]
        n1435 = call-dynamic "Set CCD_Config.vi"("error in (no error)"=w2154, "input cluster"=w2153, "Interface in"=w2149) -> ("error out"=w2155:errorcluster, "Interface out"=w2156:refnum<class "Interface.lvclass">)  [unwired: 7 in]
        n1436 = Flatten To String(anything=w2153, error in (no error)=w2154) -> (data string=w2265:string)  [unwired: 2 in, 2 out]
        n1437 = call "Write flatted cluster.vi"("error in (no error)"=w2155, "flatted cluster"=w2265, "Interface in"=w2156) -> ("error out"=w2100:errorcluster, "Interface out"=w2101:refnum<class "Interface.lvclass">)  [unwired: 7 in]
        n1438 = call "Read Exposure Time.vi"("error in (no error)"=w2100, "Interface in"=w2101) -> ("error out"=w2126:errorcluster, "Exposure Time"=w2123:dbl, "Interface out"=w2125:refnum<class "Interface.lvclass">)  [unwired: 7 in]
        n1439 = Greater Or Equal?(x=w2123, y=w2099) -> (x >= y?=w2122:bool)
        n1440 = Select(t=w2123, s=w2122, f=w2099) -> (s? t:f=w2124:dbl)
        n1441 = local write "Exptime ch4"(w2124) -> ()
        n1442 = call "Write Exposure Time.vi"("error in (no error)"=w2126, "Exposure Time"=w2124, "Interface in"=w2125) -> ("error out"=w2043:errorcluster, "Interface out"=w2048:refnum<class "Interface.lvclass">)  [unwired: 7 in]
        n1443 = call-dynamic "ValidateExp.vi"("error in (no error)"=w2043, "Interface in"=w2048) -> ("error out"=w2068:errorcluster, "Interface out"=w2047:refnum<class "Interface.lvclass">)  [unwired: 8 in]
        n1444 = call-dynamic "Read MAX #FRAMES.vi"("error in (no error)"=w2068, "Interface in"=w2047) -> ("error out"=w2069:errorcluster, "Interface out"=w2046:refnum<class "Interface.lvclass">)  [unwired: 7 in, 1 out]
        n1445 = call-dynamic "Read # Images.vi"("error in (no error)"=w2069, "Interface in"=w2046) -> ("error out"=w2067:errorcluster, "# Images"=w2040:u32, "Interface out"=w2045:refnum<class "Interface.lvclass">)  [unwired: 7 in]
        n1446 = call-dynamic "Write #PREV Images.vi"("error in (no error)"=w2067, "#PREV FRAMES"=w2040, "Interface in"=w2045) -> ("error out"=w2042:errorcluster, "Interface out"=w2044:refnum<class "Interface.lvclass">)  [unwired: 7 in]
        n1447 = local write "Exp ch4"(w2040) -> ()
        n1448 = property on="Exposures Done ch4" class="Slide (strict)"("Scale.Maximum"=w2040, "Scale.Minimum"=0.0 ("Scale.Range:Minimum")) -> ()  [unwired: 2 in, 2 out]
        n1449 = call-dynamic "Write Interface.vi"("error in (no error)"=w2042, "Interface.lvclass"=w2044, "Channel in"=w2256) -> ("error out"=w2261:errorcluster, "Channel out"=w2263:refnum<class "Channel.lvclass">)  [unwired: 7 in]
        n1450 = call "Write section_name.vi"("error in (no error)"=w2261, "section_name"="CCD_ACS4", "Channel in"=w2263) -> ("error out"=w2260:errorcluster, "Channel out"=w2262:refnum<class "Channel.lvclass">)  [unwired: 7 in]
        n1451 = call-dynamic "save config.vi"("error in (no error)"=w2260, "file config"="lastsaved.cfg", "Channel in"=w2262) -> ("error out"=w2157:errorcluster, "Channel out"=w2158:refnum<class "Channel.lvclass">)  [unwired: 7 in]
        n1452 = call-dynamic "ValidateConfig.vi"("error in (no error)"=w2157, "Channel in"=w2158) -> ("error out"=w2160:errorcluster, "Channel out"=w2161:refnum<class "Channel.lvclass">)  [unwired: 7 in, 1 out]
        n1453 = call-dynamic "Save Temp.vi"("error in (no error)"=w2160, "temp file"="lasttemp.cfg" ("file config"), "Channel in"=w2161) -> ("error out"=w2103:errorcluster, "Channel out"=w2102:refnum<class "Channel.lvclass">)  [unwired: 7 in]
        n1454 = case shown="True" w2106 {
          tunnel: [w2426 w2452] -> w2105
          tunnel: [w2427 w2451] -> w2104
          tunnel: w2103 -> [w2427 w2450]
          tunnel: w2102 -> [w2426 w2432]
          frame False {
          }
          frame True {
            # "Esvazia\na fila."
            n1455 = call-dynamic "Read State Machine.vi"("error in (no error)"=w2450, "Device in"=w2432) -> ("error out"=w2444:errorcluster, "State Machine.lvclass"=w2447:refnum<class "State Machine.lvclass">, "Device out"=w2456:refnum<class "Channel.lvclass">)  [unwired: 7 in]
            n1456 = call-dynamic "Read ref StatesQueue.vi"("error in (no error)"=w2444, "State Machine in"=w2447) -> ("error out"=w2434:errorcluster, "ref StatesQueue"=w2436:refnum<queue>, "State Machine out"=w2446:refnum<class "State Machine.lvclass">)  [unwired: 7 in]
            n1457 = Flush Queue(queue=w2436, error in (no error)=w2434) -> (queue out=w2435:refnum<queue>, error out=w2433:errorcluster)  [unwired: 1 out]
            n1458 = Enqueue Element(queue=w2435, element=u32 60 ("State"), error in (no error)=w2433) -> (queue out=w2449:refnum<queue>, error out=w2443:errorcluster)  [unwired: 1 in, 1 out]
            n1459 = Enqueue Element(queue=w2449, element=u32 45 ("State"), error in (no error)=w2443) -> (queue out=w2448:refnum<queue>, error out=w2442:errorcluster)  [unwired: 1 in, 1 out]
            n1460 = Enqueue Element(queue=w2448, element=u32 35 ("State"), error in (no error)=w2442) -> (queue out=w2441:refnum<queue>, error out=w2430:errorcluster)  [unwired: 1 in, 1 out]
            n1461 = Enqueue Element(queue=w2441, element=u32 37, error in (no error)=w2430) -> (queue out=w2431:refnum<queue>, error out=w2429:errorcluster)  [unwired: 1 in, 1 out]
            n1462 = call-dynamic "Write ref StatesQueue.vi"("error in (no error)"=w2429, "ref StatesQueue"=w2431, "State Machine in"=w2446) -> ("error out"=w2437:errorcluster, "State Machine out"=w2445:refnum<class "State Machine.lvclass">)  [unwired: 7 in]
            n1463 = disable-structure shown="Enabled" {
              disable-tunnel: [0 ("State") 45] -> w2453
              frame Enabled {
                # "Vai pra 0 para que\nos estados da fila \nsejam retirados."
              }
              frame Disabled {
                # "Verifica Texp\nantes de tudo."
              }
            }
            n1464 = call-dynamic "Write State.vi"("error in (no error)"=w2437, "State"=w2453, "State Machine in"=w2445) -> ("error out"=w2454:errorcluster, "State Machine out"=w2455:refnum<class "State Machine.lvclass">)  [unwired: 7 in]
            n1465 = call-dynamic "Write State Machine.vi"("error in (no error)"=w2454, "State Machine.lvclass"=w2455, "Device in"=w2456) -> ("error out"=w2451:errorcluster, "Device out"=w2452:refnum<class "Channel.lvclass">)  [unwired: 7 in]
          }
        }
        n1466 = call-dynamic "Write Channel.vi"("error in (no error)"=w2104, "Channel.lvclass"=w2105, "Acquisition in"=w2270) -> ("error out"=w2267:errorcluster, "Acquisition out"=w2266:refnum<class "Acquisition.lvclass">)  [unwired: 7 in]
        n1467 = call-dynamic "Write AcquisitionD.vi"("error in (no error)"=w2267, "Acquisition.lvclass"=w2266, "S4ACS_GUI in"=w2271) -> ("error out"=w2236:errorcluster, "S4ACS_GUI out"=w2239:refnum<class "S4GUI.lvclass">)  [unwired: 7 in]
        n1468 = Merge Errors(w2084, w2238, w2237, w2236) -> (w2235:errorcluster)
        n1469 = call "Write cfg file.vi"("error in (no error)"=w2235, "cfg file"="lastsaved.cfg", "S4ACS_GUI in"=w2239) -> ("error out"=w2320:errorcluster, "S4ACS_GUI out"=w2322:refnum<class "S4GUI.lvclass">)  [unwired: 7 in]
      }
      event "Frame Transfer", "AQM", "SZM", "EM Gain": Value Change {
        # "criar  S4GUI:CalcTemp.vi (metodo da classe S4GUI.lvclass)\na mesma lógica do Channel:ValidateConfig.vi usando\no cluster S4GUI:Parameters CCD em vez do cluster Interface:CCD CF.\nIgnore o Texp Min e apenas salve a temperatura em S4GUI:PrevTemp"
        # "Sinaliza que não há requisição de SET CCD mode"
        n1470 = event-data() -> ()  [unwired: 1 in, 6 out]
        n1471 = call-dynamic "Write SET request.vi"("error in (no error)"=w2514, "SET request"=FALSE, "S4GUI in"=w2516) -> ("error out"=w2513:errorcluster, "S4GUI out"=w2515:refnum<class "S4GUI.lvclass">)  [unwired: 7 in]
        n1472 = local read "Frame Transfer"() -> (w2529:enum16{"OFF", "ON"})
        n1473 = local read "EM Gain"() -> (w2518:u16)
        n1474 = local read "AQM"() -> (w2528:T4)
        n1475 = local read "SZM"() -> (w2527:T3)
        n1476 = call-dynamic "Read CCD mode.vi"("error in (no error)"=w2513, "S4GUI in"=w2515) -> ("error out"=w2526:errorcluster, "CCD mode"=w2531:T30, "S4GUI out"=w2532:refnum<class "S4GUI.lvclass">)  [unwired: 7 in]
        n1477 = Bundle By Name(cluster=w2531, "FTM"=w2529, "AQM"=w2528, "SZM"=w2527, "EM gain"=w2518) -> (w2530:T30)
        n1478 = call-dynamic "Write CCD mode.vi"("error in (no error)"=w2526, "CCD mode"=w2530, "S4GUI in"=w2532) -> ("error out"=w2524:errorcluster, "S4GUI out"=w2525:refnum<class "S4GUI.lvclass">)  [unwired: 7 in]
        n1479 = call-dynamic "LoadCCDmode.vi"("error in (no error)"=w2524, "S4GUI in"=w2525) -> ("error out"=w2522:errorcluster, "S4GUI out"=w2523:refnum<class "S4GUI.lvclass">)  [unwired: 8 in]
        n1480 = call-dynamic "Read Parameters CCD modes.vi"("error in (no error)"=w2522, "S4GUI in"=w2523) -> ("error out"=w2519:errorcluster, "Parameters CCD modes"=w2517:T5, "S4GUI out"=w2521:refnum<class "S4GUI.lvclass">)  [unwired: 7 in]
        n1481 = call-dynamic "Read InfoCCDmode.vi"("error in (no error)"=w2519, "S4GUI in"=w2521) -> ("error out"=w2509:errorcluster, "InfoCCDmode"=w2520:T2, "S4GUI out"=w2510:refnum<class "S4GUI.lvclass">)  [unwired: 7 in]
        n1482 = local write "Parameters CCD modes"(w2517) -> ()
        n1483 = local write "InfoCCDmode"(w2520) -> ()
        n1484 = call-dynamic "CalcTemp.vi"("error in (no error)"=w2509, "S4GUI in"=w2510) -> ("error out"=w2508:errorcluster, "S4GUI out"=w2507:refnum<class "S4GUI.lvclass">)  [unwired: 8 in]
        n1485 = call-dynamic "Read Prev Temp.vi"("error in (no error)"=w2508, "S4GUI in"=w2507) -> ("Prev Temp"=→"Preview Temp.":dbl)  [unwired: 7 in, 2 out]
      }
      event "TCS mode": Value Change {
        # "2024-04-04: Não se usa mais o ID para configurar a comunicação..."
        # "simul"
